vi "E15_Máquina de esados.vi"() -> ()   [LabVIEW 2026]
panel:
  out "String":string
  in  "stop":bool
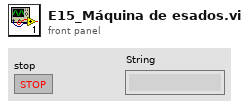
[diagram p1: front panel]
types:
  T1 = enum16{"Inicio", "Paso 1", "Paso 2", "Paso 3", "Finalizar"}
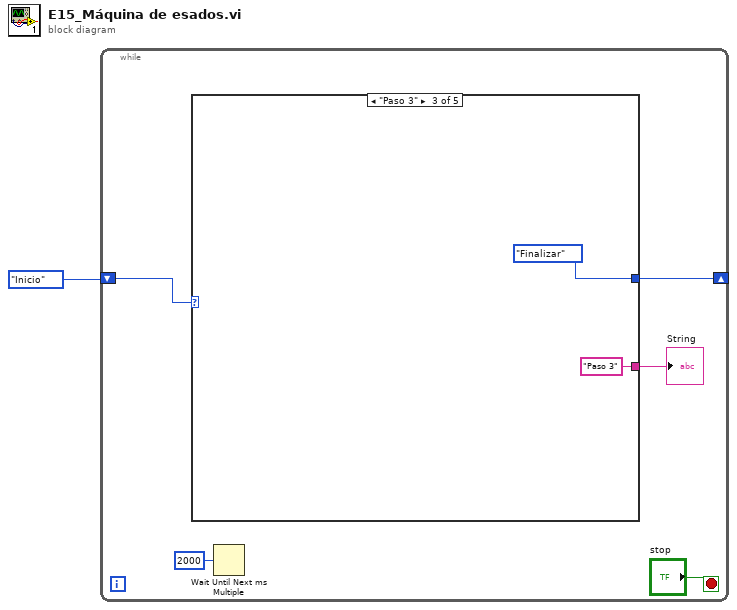
[diagram p0: block diagram]
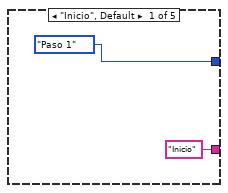
[diagram p2: hidden frame]
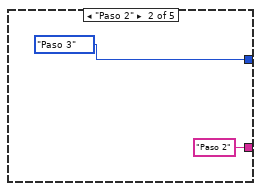
[diagram p3: hidden frame]
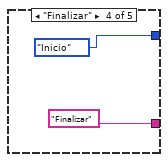
[diagram p4: hidden frame]
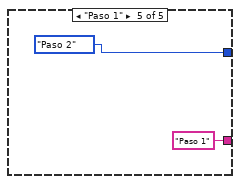
[diagram p5: hidden frame]
diagram:
  n1 = while {
    shift-right: [w3] -> _
    shift-left: T1."Inicio" -> [w4]
    stop <- "stop" stop-if-true
    n2 = case shown="\"Paso 3\"" w4 {
      tunnel: ["Inicio" "Paso 2" "Paso 3" "Finalizar" "Paso 1"] -> w5
      tunnel: [T1."Paso 1" T1."Paso 3" T1."Finalizar" T1."Inicio" T1."Paso 2"] -> w3
      frame "Inicio", Default {
      }
      frame "Paso 2" {
      }
      frame "Paso 3" {
      }
      frame "Finalizar" {
      }
      frame "Paso 1" {
      }
    }
    "String" <- w5
    n3 = Wait Until Next ms Multiple(millisecond multiple=u32 2000) -> ()  [unwired: 1 out]
  }
